vi "Actor Core.vi"(8 "error in":errorcluster, 11 "ActorBlockedUntilNotified in":refnum<class "ActorBlockedUntilNotified.lvclass">) -> (0 "error out":errorcluster, 3 "Actor out":refnum<class "Actor.lvclass">)   [LabVIEW 2017, in "ActorBlockedUntilNotified.lvclass"]
doc: "(<B>Filename</B>: Actor Framework.lvlib:Actor.lvclass:Actor Core.vi)\n\nReceives messages to the actor, reacts to them, and initiates any error handling that may shut the actor down.\n\nDescendant classes may override this VI to append parallel tasks for the actor to complete while it handles messages. Overrides use the Call Parent Method node."
uses:
  ActorBlockedUntilNotified.lvclass
  C:/Program Files (x86)/National Instruments/LabVIEW 2017/vi.lib/ActorFramework/Actor/Actor.lvclass
  <vilib>/ActorFramework/Actor/Actor.lvclass
  <vilib>/ActorFramework/Actor/Actor.lvclass/Actor.ctl
  <vilib>/ActorFramework/Message Enqueuer/Message Enqueuer.lvclass/Message Enqueuer.ctl
  ActorBlockedUntilNotified.lvclass/ActorBlockedUntilNotified.ctl
  <vilib>/ActorFramework/Stop Msg/Stop Msg.lvclass/Stop Msg.ctl
  <vilib>/ActorFramework/Message Enqueuer/Init from Existing Queue.vi
  <vilib>/ActorFramework/Message Enqueuer/Enqueue Critical.vi
  <vilib>/ActorFramework/Stop Msg/Stop Msg.lvclass
  C:/Program Files (x86)/National Instruments/LabVIEW 2017/vi.lib/ActorFramework/Message/Message.lvclass
  <vilib>/ActorFramework/Message Priority Queue/Priority Enqueue.vi
  <vilib>/ActorFramework/Message Enqueuer/Message Enqueuer.lvclass
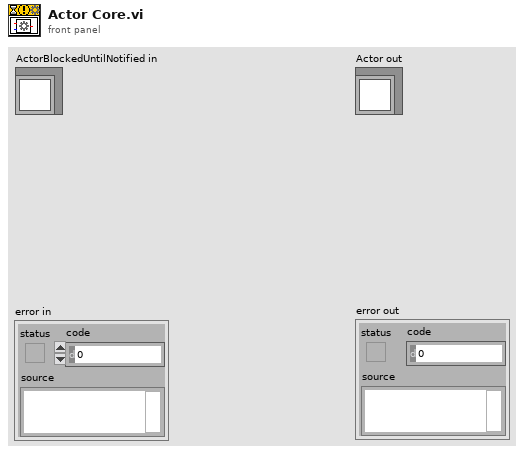
[diagram p1: front panel]
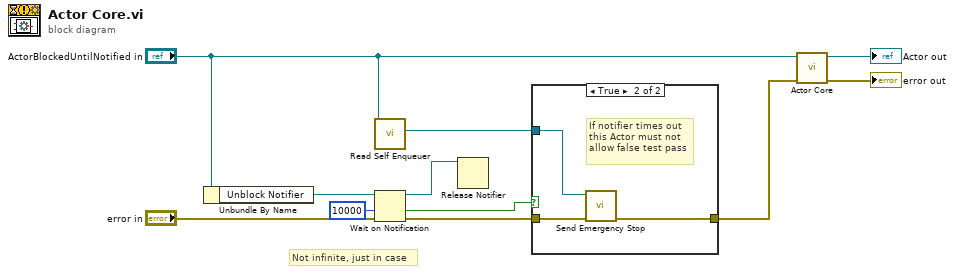
[diagram p0: block diagram]
diagram:
  # "Not infinite, just in case"
  n1 = Unbundle By Name("ActorBlockedUntilNotified in") -> ("Unblock Notifier"=w8:refnum<notifier>)
  n2 = call <vilib>:"Read Self Enqueuer.vi"("Actor"="ActorBlockedUntilNotified in") -> ("Self Enqueuer"=w5:refnum<class "Message Enqueuer.lvclass">)  [unwired: 10 in]
  n3 = Wait on Notification(notifier=w8, timeout in ms (-1)=10000, error in (no error)="error in") -> (notifier out=w1:refnum<notifier>, timed out?=w2:bool, error out=w4:errorcluster)  [unwired: 1 in, 1 out]
  n4 = Release Notifier(notifier=w1) -> ()  [unwired: 2 in, 3 out]
  n5 = case shown="True" w2 {
    tunnel: w5 -> [_ w15]
    tunnel: w4 -> [w12 w14]
    tunnel: [w12 w13] -> w3
    frame False {
      # "Carry on!"
    }
    frame True {
      # "If notifier times out\nthis Actor must not\nallow false test pass"
      n6 = call <vilib>:"Send Emergency Stop.vi"("error in (no error)"=w14, "Message Enqueuer"=w15) -> ("error out"=w13:errorcluster)  [unwired: 9 in]
    }
  }
  n7 = call-parent "Actor Core.vi"("error in"=w3, "Actor in"="ActorBlockedUntilNotified in") -> ("error out"=→"error out":errorcluster, "Actor out"=→"Actor out":refnum<class "Actor.lvclass">)  [unwired: 8 in]
